vi "FTW-Benchmark-JSON-Number-Parse.vi"() -> ()   [LabVIEW 2015]
uses:
  source/JSON/FTW-JSON-Part.ctl
  source/JSON/FTW-JSON-LexicalScan.ctl
panel:
  in  "format string":string="%_17e"
  out "Improvement":dbl format="%.1f %"
  in  "Parallel Instances":i32=8
  out "error out":errorcluster
  out "Results":T1(array[cluster])
  out "Lexical Parser Time":dbl format="%.3ps"
  out "Regex Parser Time":dbl format="%.3ps"
  in  "Unique Numbers":i32=10000
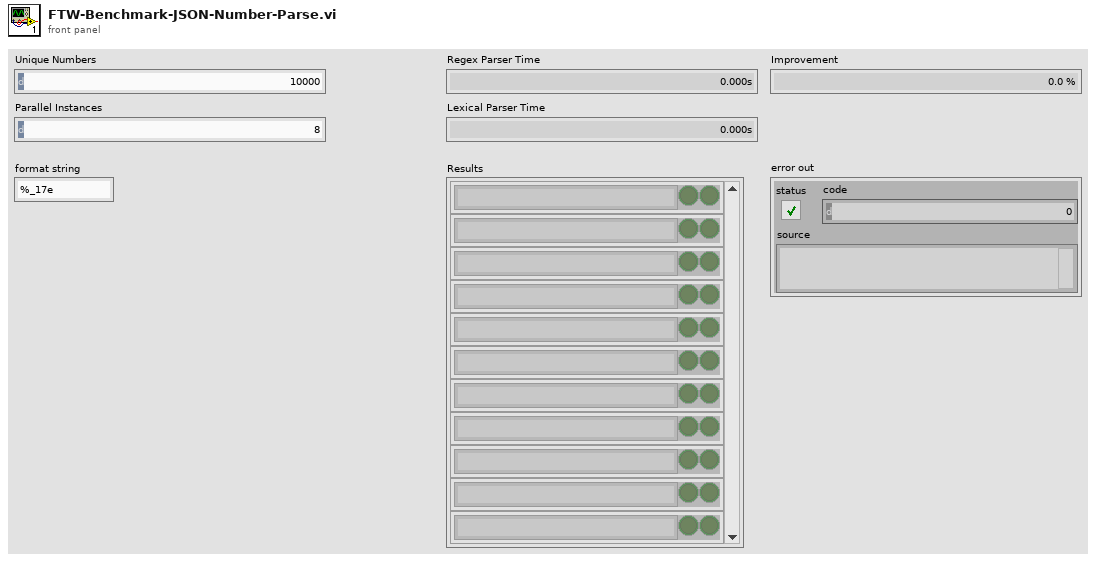
[diagram p1: front panel]
types:
  T1 = cluster{string, "Status OK?":bool, "Status OK?":bool}[]
  T2 = typedef "FTW-JSON-Part.ctl" = enum8{"Not Found", "Object", "Object Inner", "Array", "Array Inner", "String", "Number", "Boolean", "null"}
  T3 = typedef "FTW-JSON-LexicalScan.ctl" = cluster{"String":string, "Position":i32, "Line":i32, "Column":i32}
  T4 = cluster{string, "Status OK?":bool, "Status OK?":bool}
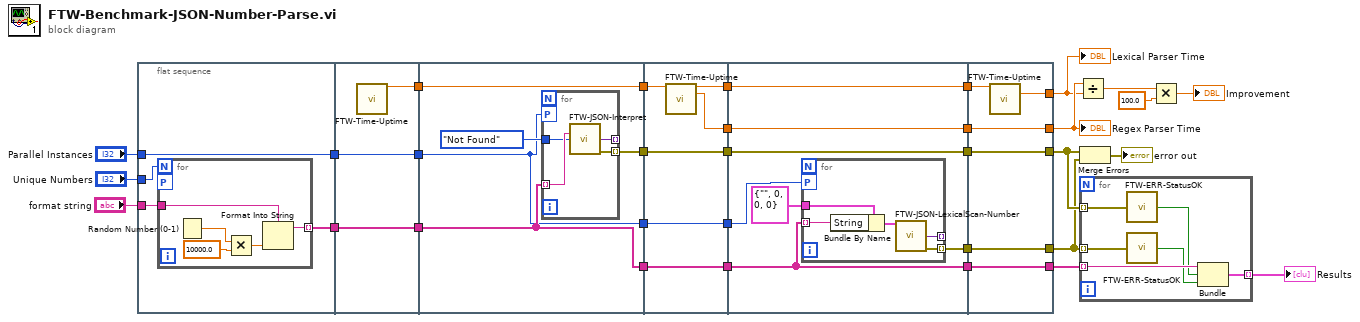
[diagram p0: block diagram]
diagram:
  n1 = flat-sequence {
    tunnel: "Unique Numbers" -> [w36]
    tunnel: [w35] -> w31
    tunnel: [w34] -> w10
    tunnel: "Parallel Instances" -> [w34]
    tunnel: "format string" -> [w33]
    tunnel: w31 -> [w43]
    tunnel: [w44] -> w30
    tunnel: [w43] -> w29
    tunnel: [w42] -> w11
    tunnel: w10 -> [w42]
    tunnel: w30 -> [w49]
    tunnel: w29 -> [w48]
    tunnel: [w49] -> w28
    tunnel: [w48] -> w27
    tunnel: [w46] -> w26
    tunnel: w11 -> [w45]
    tunnel: [w45] -> w7
    tunnel: w28 -> [w59]
    tunnel: w27 -> [w58]
    tunnel: w26 -> [w57]
    tunnel: [w56] -> w25
    tunnel: [w58] -> w24
    tunnel: [w57] -> w23
    tunnel: [w55] -> w13
    tunnel: [w54] -> w8
    tunnel: w7 -> [w54]
    tunnel: w25 -> [w66]
    tunnel: w24 -> [w64]
    tunnel: w23 -> [w65]
    tunnel: [w66] -> w22
    tunnel: [w64] -> w21
    tunnel: [w65] -> w20
    tunnel: [w63] -> w19
    tunnel: w13 -> [w61]
    tunnel: [w61] -> w12
    tunnel: w8 -> [w60]
    tunnel: [w75] -> w16
    tunnel: [w76] -> w18
    tunnel: [w74] -> w5
    tunnel: w22 -> [w77]
    tunnel: w21 -> [w76]
    tunnel: w20 -> [w75]
    tunnel: [w73] -> w15
    tunnel: w19 -> [w73]
    tunnel: w12 -> [w72]
    tunnel: [w72] -> w6
    frame #0 {
      n2 = for {
        N: w36 -> [_]
        tunnel: [w38] -> w35 mode=indexing
        workers-P: _ -> [_]
        tunnel: w33 -> [w37]
        n3 = Random Number (0-1)() -> (number: 0 to 1=w41:dbl)
        n4 = Multiply(x=w41, y=10000.0) -> (x*y=w39:dbl)
        n5 = Format Into String(format string=w37, w39) -> (resulting string=w38:string)  [unwired: 2 in, 1 out]
      }
    }
    frame #1 {
      n6 = call "FTW-Time-Uptime.vi"() -> ("Current Uptime"=w44:dbl)  [unwired: 13 in, 2 out]
    }
    frame #2 {
      n7 = for {
        tunnel: w48 -> [w53] mode=indexing
        tunnel: FTW-JSON-Part."Not Found" ("JSON Parent") -> [w52]
        tunnel: [w51] -> w46 mode=indexing
        tunnel: [w50] -> _ mode=indexing
        workers-P: w45 -> [_]
        n8 = call "FTW-JSON-Interpret.vi"("JSON String"=w53, "JSON Parent"=w52) -> ("Container"=w50:variant, "error out"=w51:errorcluster)  [unwired: 8 in, 4 out]
      }
    }
    frame #3 {
      n9 = call "FTW-Time-Uptime.vi"("Previous Uptime"=w59) -> ("Current Uptime"=w56:dbl, "Elapsed Time"=w55:dbl)  [unwired: 12 in, 1 out]
    }
    frame #4 {
      n10 = for {
        tunnel: w64 -> [w69] mode=indexing
        tunnel: [w68] -> w63 mode=indexing
        tunnel: T3 {"String"="", "Position"=0, "Line"=0, "Column"=0} ("JSON String") -> [w71]
        tunnel: [w67] -> _ mode=indexing
        workers-P: w60 -> [_]
        n11 = Bundle By Name(cluster=w71, "String"=w69) -> (w70:T3)
        n12 = call "FTW-JSON-LexicalScan-Number.vi"("JSON String"=w70) -> ("Number"=w67:variant, "error out"=w68:errorcluster)  [unwired: 12 in, 1 out]
      }
    }
    frame #5 {
      n13 = call "FTW-Time-Uptime.vi"("Previous Uptime"=w77) -> ("Elapsed Time"=w74:dbl)  [unwired: 12 in, 2 out]
    }
  }
  n14 = Divide(x=w6, y=w5) -> (x/y=w4:dbl)
  n15 = Merge Errors(w16, w15) -> (→"error out":errorcluster)
  n16 = for {
    tunnel: w18 -> [w83] mode=indexing
    tunnel: w16 -> [w82] mode=indexing
    tunnel: w15 -> [w81] mode=indexing
    tunnel: [w78] -> w17 mode=indexing
    n17 = call "FTW-ERR-StatusOK.vi"("error to check"=w82) -> ("Status OK?"=w80:bool)
    n18 = call "FTW-ERR-StatusOK.vi"("error to check"=w81) -> ("Status OK?"=w79:bool)
    n19 = Bundle(w83, "Status OK?"=w80, "Status OK?"=w79) -> (w78:T4)  [unwired: 1 in]
  }
  "Results" <- w17
  n20 = Multiply(x=w4, y=100.0 ("x")) -> (x*y=→"Improvement":dbl)
  "Lexical Parser Time" <- w5
  "Regex Parser Time" <- w6
